vi "WriteConfiguration.vi"(10 "Content":string="[LVUnit]\nProjectLibrarySuffix=Test.lvlib\nDeferDrawingDuringTest=True") -> (0 "error out":errorcluster)   [LabVIEW 2017, in "Configuration.Tests.lvlib"]
uses:
  Configuration.Tests.lvlib
  Configuration/Configuration.lvlib
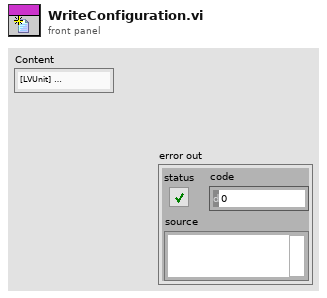
[diagram p1: front panel]
types:
  T1 = enum16{"open", "replace", "create", "open or create", "replace or create", "replace or create with confirmation"}
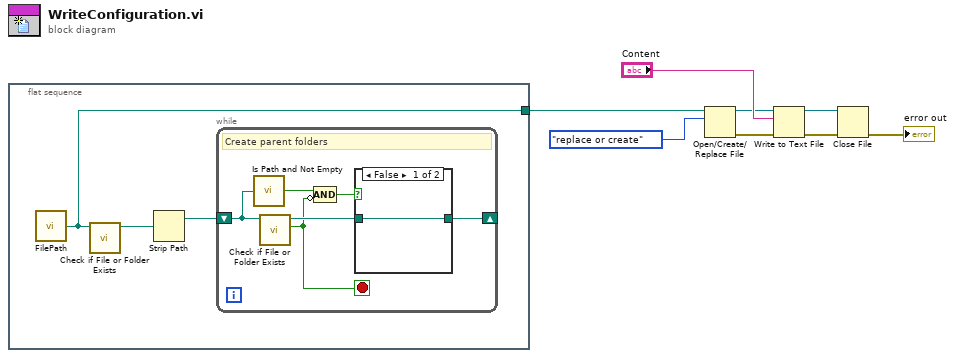
[diagram p0: block diagram]
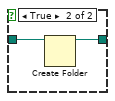
[diagram p2: hidden frame]
diagram:
  n1 = flat-sequence {
    tunnel: [w9] -> w1
    frame #0 {
      n2 = call "FilePath.vi"() -> ("File Path"=w9:path)
      n3 = call <vilib>:"Check if File or Folder Exists.vi"("path"=w9) -> ("dup path"=w11:path)  [unwired: 8 in, 2 out]
      n4 = Strip Path(path=w11) -> (stripped path=w10:path)  [unwired: 1 out]
      n5 = while {
        shift-right: [w13] -> _
        shift-left: w10 -> [w17]
        stop <- w12 stop-if-true
        # "Create parent folders"
        n6 = call <vilib>:"Is Path and Not Empty.vi"("path"=w17) -> ("Is Path and Not Empty?"=w16:bool)  [unwired: 4 in]
        n7 = call <vilib>:"Check if File or Folder Exists.vi"("path"=w17) -> ("file or folder exists?"=w12:bool, "dup path"=w15:path)  [unwired: 8 in, 1 out]
        n8 = Compound Arithmetic op=AND(w16, invert w12) -> (w14:bool)
        n9 = case shown="False" w14 {
          tunnel: w15 -> [w18 w20]
          tunnel: [w18 w19] -> w13
          frame False {
          }
          frame True {
            n10 = Create Folder(path (use dialog)=w20) -> (created path=w19:path)  [unwired: 2 in, 2 out]
          }
        }
      }
    }
  }
  n11 = Open/Create/Replace File(file path (use dialog)=w1, operation (0:open)=T1."replace or create") -> (refnum out=w3:refnum<file>, error out=w4:errorcluster)  [unwired: 4 in, 1 out]
  n12 = Write to Text File(file (use dialog)=w3, text="Content", error in=w4) -> (refnum out=w6:refnum<file>, error out=w7:errorcluster)  [unwired: 1 in, 1 out]
  n13 = Close File(refnum=w6, error in=w7) -> (error out=→"error out":errorcluster)  [unwired: 1 out]
